vi "Read Color.vi"(11 "Game Board Component in":refnum<class "Game Board Component.lvclass">) -> (2 "color":u32(colorbox))   [LabVIEW 2021, in "Game Board Component.lvclass"]
doc: "MIT Licence\nCopyright (c) 2024 David Grollier"
uses:
  Game Board Component.lvclass
  Game Board Component.lvclass/Game Board Component.ctl
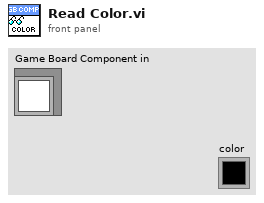
[diagram p1: front panel]
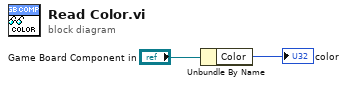
[diagram p0: block diagram]
diagram:
  n1 = Unbundle By Name("Game Board Component in") -> ("Color"=→"color":u32)
